vi "Check EXT Range.vi"(9 "EXT Value":ext, 11 "EXT Control":refnum<vi>) -> (1 "In Range?":bool, 3 "Coerced Range":ext)   [LabVIEW 2024]
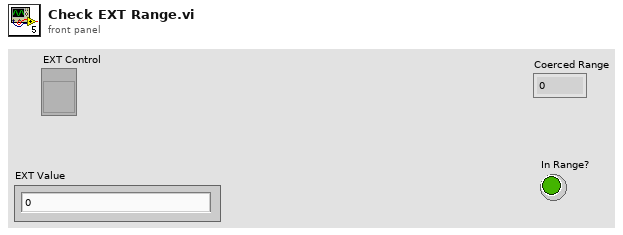
[diagram p1: front panel]
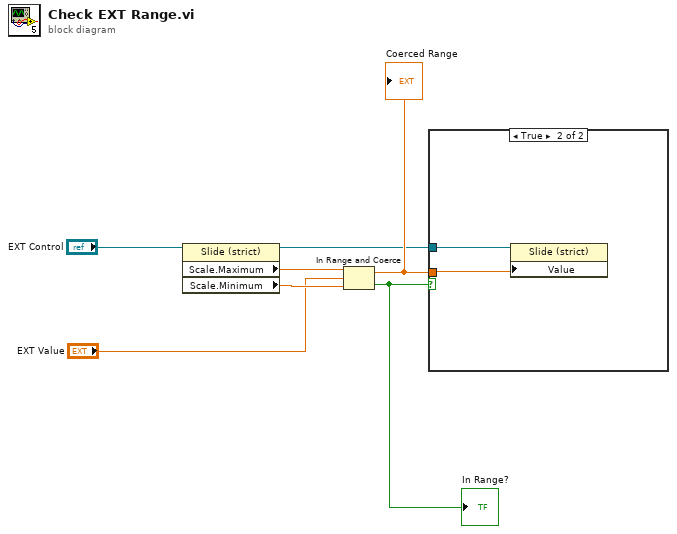
[diagram p0: block diagram]
diagram:
  n1 = property class="Slide (strict)"(reference="EXT Control") -> (reference out=w2:refnum<vi>, "Scale.Maximum"=w7:dbl, "Scale.Minimum"=w6:dbl)  [unwired: 1 in, 1 out]
  n2 = In Range and Coerce(upper limit=w7, x="EXT Value", lower limit=w6) -> (coerced(x)=w3:ext, In Range?=w1:bool)
  "In Range?" <- w1
  "Coerced Range" <- w3
  n3 = case shown="True" w1 {
    tunnel: w3 -> [_ w8]
    tunnel: w2 -> [_ w9]
    frame False {
    }
    frame True {
      n4 = property class="Slide (strict)"(reference=w9, "Value"=w8) -> ()  [unwired: 1 in, 2 out]
    }
  }
